vi "Delacor_lib_QMH_DQMH Error Tags--constant.vi"() -> (1 "Close Tag":string, 3 "Open Tag":string)   [LabVIEW 2024, in "JQMH_Message Queue.lvclass"]
doc: "____\nDQMH Framework: Palette 7.1.0.1503\nCopyright (c) 2025, DQMH Consortium"
uses:
  JQMH_Message Queue.lvclass
  JQMH_Message Queue.lvclass/JQMH_Message Queue.ctl
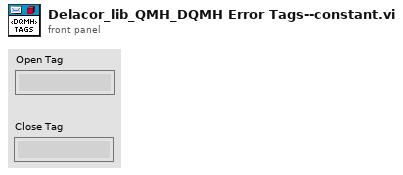
[diagram p1: front panel]
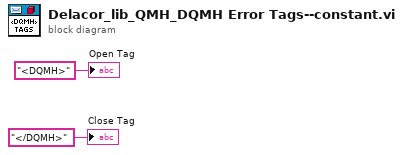
[diagram p0: block diagram]
diagram:
  "Open Tag" <- "<DQMH>" ("Open Tag")
  "Close Tag" <- "</DQMH>" ("Close Tag")
